vi "getRange.vi"(8 "error in (no error)":errorcluster, 11 "AoDeviceData in":refnum<class "AoDeviceData.lvclass">) -> (0 "error out":errorcluster, 1 "max":dbl, 2 "min":dbl, 3 "AoDeviceData out":refnum<class "AoDeviceData.lvclass">)   [LabVIEW 2011, in "DataMappers.lvlib" / "AoDeviceData.lvclass"]
uses:
  AoDeviceData.lvclass
  DatabaseHelpers/Database Objects/device/AnalogDevice/AnalogDevice.lvclass
  DeviceData.lvclass
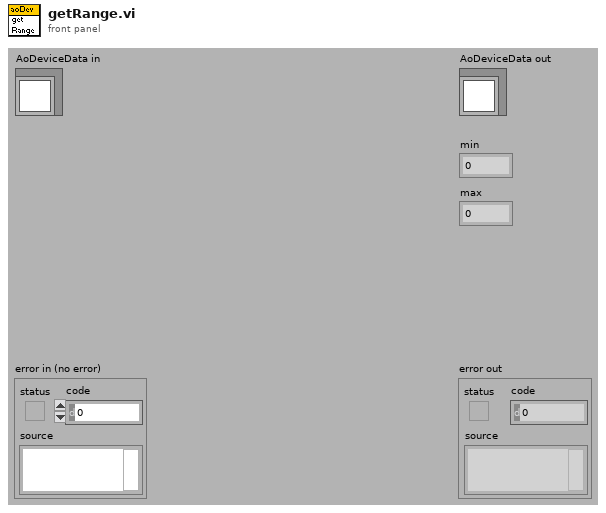
[diagram p1: front panel]
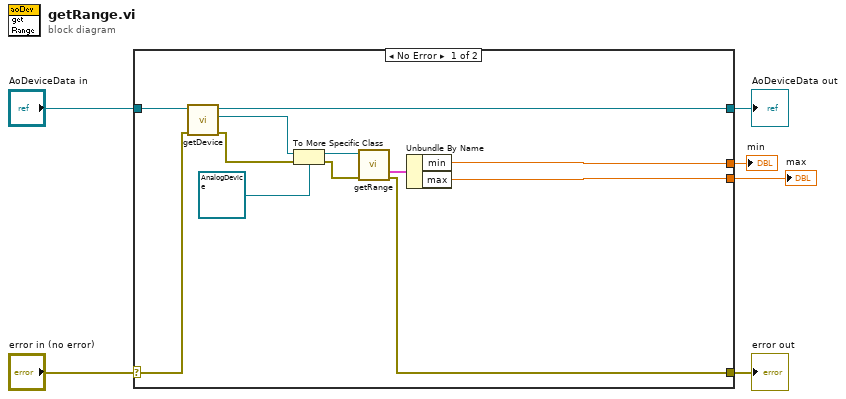
[diagram p0: block diagram]
diagram:
  n1 = case shown="No Error" "error in (no error)" {
    selector: "error in (no error)" -> [w16 w20]
    tunnel: [w7 w20] -> w5
    tunnel: [w17 w19] -> w3
    tunnel: "AoDeviceData in" -> [w18 w19]
    tunnel: [w9 _] -> w2
    tunnel: [w8 _] -> w1
    frame No Error {
      n2 = call "getDevice.vi"("error in (no error)"=w16, "DeviceData.lvclass in"=w18) -> ("error out"=w13:errorcluster, "device"=w14:refnum<class "device.lvclass">, "DeviceData.lvclass out"=w17:refnum<class "AoDeviceData.lvclass">)  [unwired: 7 in]
      n3 = To More Specific Class(target class=refnum<class "AnalogDevice.lvclass"> refnum ("Tools.lvlib:DatabaseHelpers.lvlib:AnalogDevice.lvclass"), reference=w14, error in=w13) -> (specific class reference=w12:refnum<class "AnalogDevice.lvclass">, error out=w11:errorcluster)
      n4 = call "getRange.vi"("error in (no error)"=w11, "AnalogDevice.lvclass in"=w12) -> ("error out"=w7:errorcluster, "Range"=w10:cluster{"units":string, "min":dbl, "max":dbl})  [unwired: 7 in, 1 out]
      n5 = Unbundle By Name(w10) -> ("min"=w9:dbl, "max"=w8:dbl)
    }
    frame Error {
    }
  }
  "error out" <- w5
  "AoDeviceData out" <- w3
  "min" <- w2
  "max" <- w1
